vi "Scroller_FGGA_Pump.vi"() -> ()   [LabVIEW 2014]
uses:
  <vilib>/Instr/_visa.llb/VISA Set IO Buffer Mask.ctl
  <vilib>/Instr/_visa.llb/VISA Configure Serial Port (Instr).vi
panel:
  out "element":string
  out "Measured Motor Power (W)":dbl(knob) scale=0.0..800.0
  out "Measured Link Voltage (V)":dbl(knob) scale=0.0..800.0
  out "Measured Motor Current (A)":dbl(knob) scale=0.0..6.0
  out "Pump Controller Temperature":i32(slide) scale=0.0..100.0
  out "Pump Temperature":i32(slide) scale=-500.0..100.0
  in  "Standby Speed threshold":u32(slide) scale=66.0..100.0
  out "Array":string[](array[string])
  in  "Normal Speed threshold":u32(slide) scale=50.0..100.0
  out "running?":bool
  out "Loop Count":i32
  out "Fault register":bool[](array[boolean])
  out "Warning register":bool[](array[boolean])
  out "System status register 2":bool[](array[boolean])
  out "System status register":bool[](array[boolean])
  out "Motor Frequency":i32(graph)
  in  "Set AutoRun":bool
  in  "stop":bool
  in  "Use Standby Speed":bool
  out "error out":errorcluster
  out "Data Out":string
  in  "VISA resource name":refnum<visa-resource-name>="ASRL10::INSTR"
  in  "Pump On/Off":bool
  # "Power limit is active"
  # "Stop command received and pump is stopping"
  # "Acceleration is limited"
  # "Accelerating / running"
  # "Standby Active"
  # "Deceleration is limited"
  # "Above normal speed"
  # "Operating above the ramp speed threshold"
  # "Operating above the overload speed threshold"
  # "Warning Condition"
  # "Control mode"
  # "Fault Condition"
  # "Serial enable active"
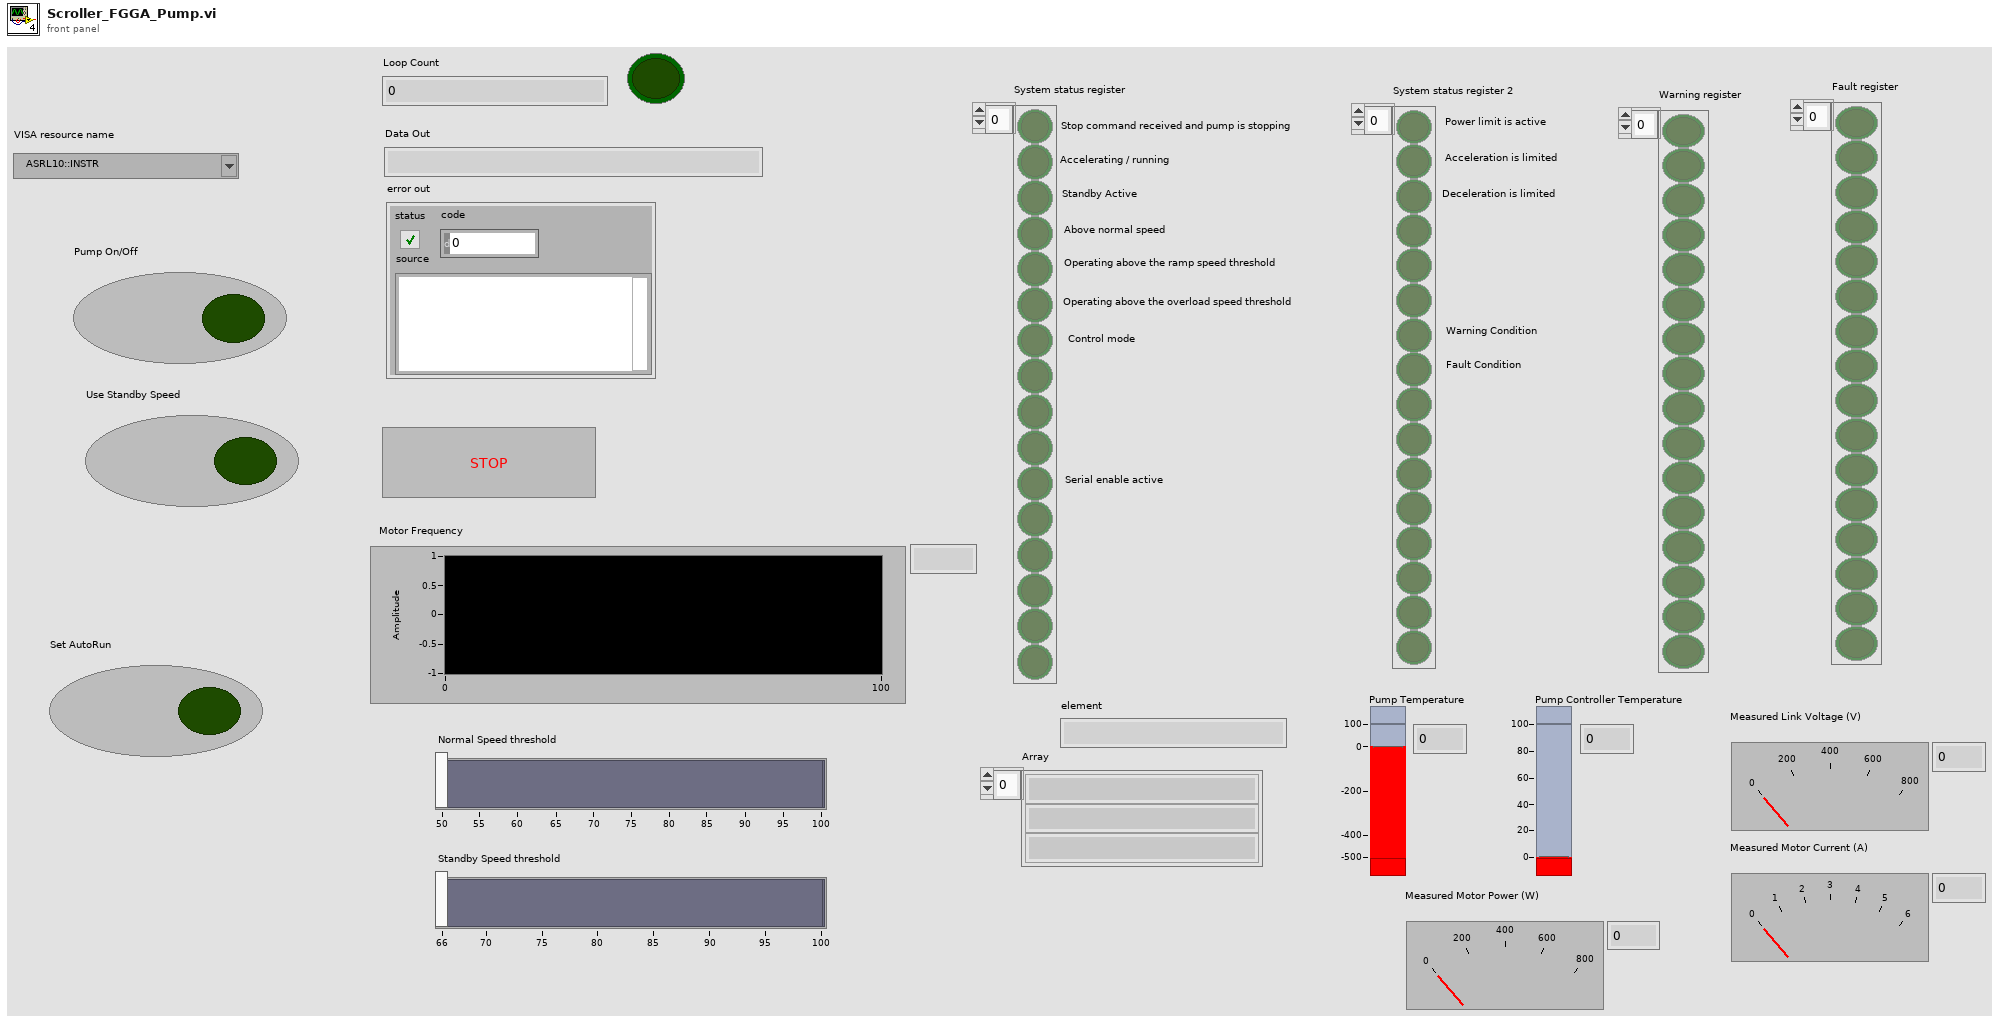
[diagram p1: front panel]
types:
  T1 = typedef "VISA Set IO Buffer Mask.ctl" = u16
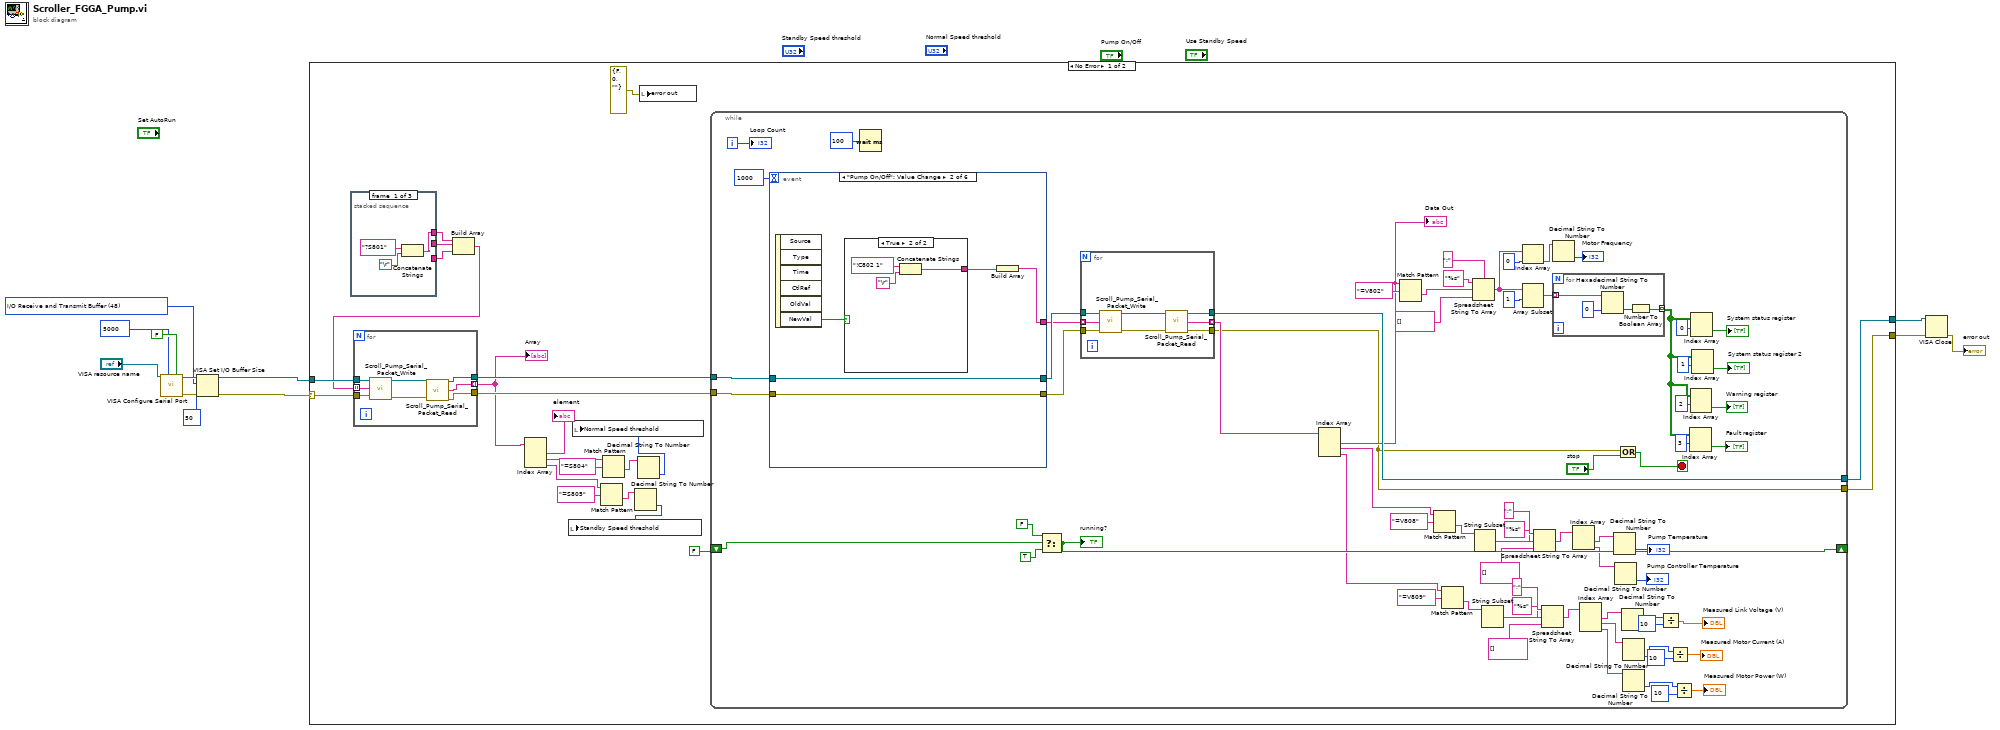
[diagram p0: block diagram]
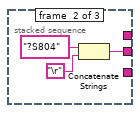
[diagram p2: hidden frame]
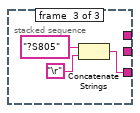
[diagram p3: hidden frame]
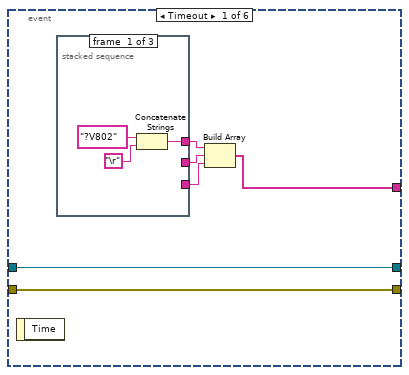
[diagram p4: hidden frame]
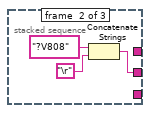
[diagram p5: hidden frame]
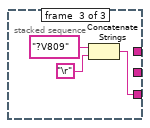
[diagram p6: hidden frame]
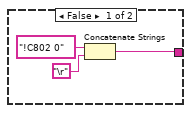
[diagram p7: hidden frame]
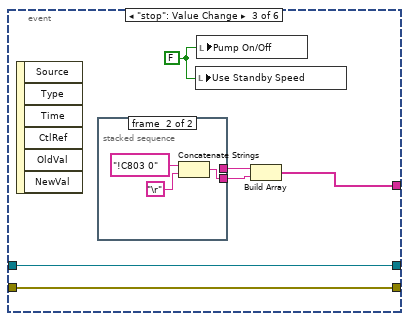
[diagram p8: hidden frame]
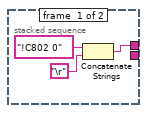
[diagram p9: hidden frame]
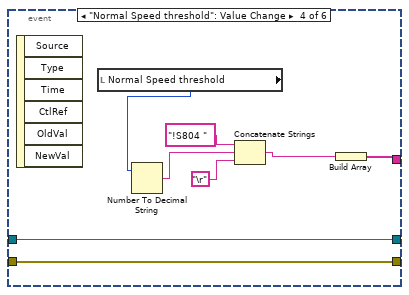
[diagram p10: hidden frame]
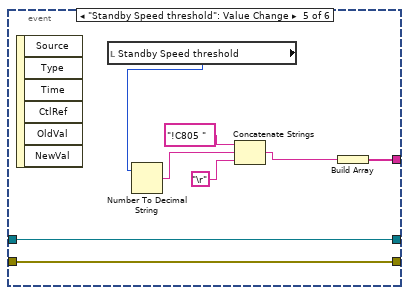
[diagram p11: hidden frame]
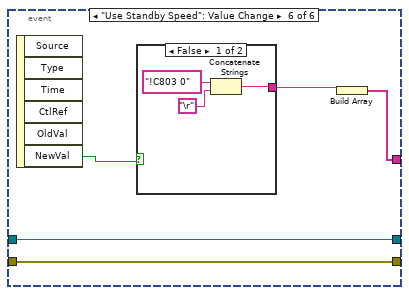
[diagram p12: hidden frame]
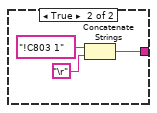
[diagram p13: hidden frame]
diagram:
  w8 = T1 48 items=["I/O Receive Buffer"=16, "I/O Transmit Buffer"=32, "I/O Receive and Transmit Buffer"=48] ("Mask")
  n1 = call-poly "VISA Configure Serial Port"("VISA resource name"="VISA resource name", "timeout (10sec)"=u32 5000, "Enable Termination\nChar (T)"=FALSE ("Enable Termination\nChar (T)")) -> ("VISA resource name out"=w9:refnum<visa-resource-name>, "error out"=w10:errorcluster)  [unwired: 11 in]
  n2 = VISA Set I/O Buffer Size(VISA resource name=w9, mask (16)=w8, size (4096)=u32 50, error in (no error)=w10) -> (VISA resource name out=w2:refnum<visa-resource-name>, error out=w1:errorcluster)
  n3 = case shown="No Error" w1 {
    selector: w1 -> [w32 w199]
    tunnel: w2 -> [w33 w200]
    tunnel: [w29 w200] -> w5
    tunnel: [w28 w199] -> w4
    frame No Error {
      n4 = stacked-sequence {
        tunnel: [_ w46 _] -> w26
        tunnel: [_ _ w49] -> w25
        tunnel: [w43 _ _] -> w23
        frame #0 {
          n5 = Concatenate Strings("?S801" ("string"), "\r") -> (w43:string)
        }
        frame #1 {
          n6 = Concatenate Strings("?S804" ("string"), "\r") -> (w46:string)
        }
        frame #2 {
          n7 = Concatenate Strings("?S805" ("string"), "\r") -> (w49:string)
        }
      }
      n8 = Build Array(w23, w26, w25) -> (w24:string[])
      n9 = for {
        tunnel: w33 -> [w42]
        tunnel: w32 -> [w41]
        tunnel: w24 -> [w40] mode=indexing
        tunnel: [w39] -> w31
        tunnel: [w38] -> w30
        tunnel: [w37] -> w17 mode=indexing
        n10 = call "Scroll_Pump_Serial_Packet_Write.vi"("VISA resource name In"=w42, "Data in"=w40, "error in (no error)"=w41) -> ("VISA resource name Out"=w36:refnum<visa-resource-name>, "error out"=w35:errorcluster)  [unwired: 11 in]
        n11 = call "Scroll_Pump_Serial_Packet_Read.vi"("VISA resource In"=w36, "error in"=w35) -> ("VISA resource Out"=w38:refnum<visa-resource-name>, "Data Out"=w37:string, "error out"=w39:errorcluster)  [unwired: 11 in]
      }
      "Array" <- w17
      n12 = Index Array(array=w17) -> (element #1=→"element":string, element #2=w22:string, element #3=w19:string)  [unwired: 3 in]
      n13 = Match Pattern(string=w19, regular expression="=S805") -> (after substring=w16:string)  [unwired: 1 in, 3 out]
      n14 = Match Pattern(string=w22, regular expression="=S804") -> (after substring=w18:string)  [unwired: 1 in, 3 out]
      n15 = Decimal String To Number(string=w16) -> (number=w14:i32)  [unwired: 2 in, 1 out]
      n16 = local write "Standby Speed threshold"(w14) -> ()
      n17 = Decimal String To Number(string=w18) -> (number=w15:i32)  [unwired: 2 in, 1 out]
      n18 = local write "Normal Speed threshold"(w15) -> ()
      n19 = local write "error out"(errorcluster {"status"=FALSE, "code"=0, "source"=""} ("error out 2")) -> ()
      n20 = while {
        shift-right: [w114] -> _
        shift-left: FALSE -> [w117]
        tunnel: w31 -> [w113]
        tunnel: w30 -> [w112]
        tunnel: [w111] -> w29
        tunnel: [w54] -> w28
        i -> [w118]
        stop <- w53 stop-if-true
        n21 = event shown="[1] \"Pump On/Off\": Value Change" {
          selector: _ -> [_ _ _ _ _ _]
          dyn-events: _ -> [_ _ _ _ _ _]
          timeout: 1000 -> [_ _ _ _ _ _]
          tunnel: [w138 w151 w161 w175 w184 w190] -> w120
          tunnel: [w137 w152 w160 w174 w183 w191] -> w119
          tunnel: w113 -> [w137 w152 w160 w174 w183 w191]
          tunnel: w112 -> [w138 w151 w161 w175 w184 w190]
          tunnel: [w139 w149 w162 w172 w180 w188] -> w60
          event Timeout {
            n22 = event-data() -> ()  [unwired: 1 in, 1 out]
            n23 = stacked-sequence {
              tunnel: [w140 _ _] -> w136
              tunnel: [_ w143 _] -> w135
              tunnel: [_ _ w146] -> w134
              frame #0 {
                n24 = Concatenate Strings("?V802" ("string"), "\r") -> (w140:string)
              }
              frame #1 {
                n25 = Concatenate Strings("?V808" ("string"), "\r") -> (w143:string)
              }
              frame #2 {
                n26 = Concatenate Strings("?V809" ("string"), "\r") -> (w146:string)
              }
            }
            n27 = Build Array(w136, w135, w134) -> (w139:string[])
          }
          event "Pump On/Off": Value Change {
            n28 = event-data() -> ("NewVal"=w153:bool)  [unwired: 1 in, 5 out]
            n29 = case shown="True" w153 {
              tunnel: [w154 w157] -> w150
              frame False {
                n30 = Concatenate Strings("!C802 0" ("string"), "\r") -> (w154:string)
              }
              frame True {
                n31 = Concatenate Strings("!C802 1" ("string"), "\r") -> (w157:string)
              }
            }
            n32 = Build Array(w150) -> (w149:string[])
          }
          event "stop": Value Change {
            w165 = FALSE
            n33 = event-data() -> ()  [unwired: 1 in, 6 out]
            n34 = stacked-sequence {
              tunnel: [w166 _] -> w164
              tunnel: [_ w169] -> w163
              frame #0 {
                n35 = Concatenate Strings("!C802 0" ("string"), "\r") -> (w166:string)
              }
              frame #1 {
                n36 = Concatenate Strings("!C803 0" ("string"), "\r") -> (w169:string)
              }
            }
            n37 = local write "Use Standby Speed"(w165) -> ()
            n38 = local write "Pump On/Off"(w165) -> ()
            n39 = Build Array(w164, w163) -> (w162:string[])
          }
          event "Normal Speed threshold": Value Change {
            n40 = event-data() -> ()  [unwired: 1 in, 6 out]
            n41 = local read "Normal Speed threshold"() -> (w177:u32)
            n42 = Number To Decimal String(number=w177) -> (decimal integer string=w176:string)  [unwired: 1 in]
            n43 = Concatenate Strings("!S804 " ("string"), w176, "\r") -> (w173:string)
            n44 = Build Array(w173) -> (w172:string[])
          }
          event "Standby Speed threshold": Value Change {
            n45 = event-data() -> ()  [unwired: 1 in, 6 out]
            n46 = local read "Standby Speed threshold"() -> (w182:u32)
            n47 = Number To Decimal String(number=w182) -> (decimal integer string=w185:string)  [unwired: 1 in]
            n48 = Concatenate Strings("!C805 " ("string"), w185, "\r") -> (w181:string)
            n49 = Build Array(w181) -> (w180:string[])
          }
          event "Use Standby Speed": Value Change {
            n50 = event-data() -> ("NewVal"=w192:bool)  [unwired: 1 in, 5 out]
            n51 = case shown="False" w192 {
              tunnel: [w193 w196] -> w189
              frame False {
                n52 = Concatenate Strings("!C803 0" ("string"), "\r") -> (w193:string)
              }
              frame True {
                n53 = Concatenate Strings("!C803 1" ("string"), "\r") -> (w196:string)
              }
            }
            n54 = Build Array(w189) -> (w188:string[])
          }
        }
        n55 = Wait (ms)(milliseconds to wait=u32 100) -> ()  [unwired: 1 out]
        n56 = Select(t=FALSE, s=w117, f=TRUE) -> (s? t:f=w114:bool)
        "running?" <- w114
        n57 = for {
          tunnel: [w127] -> w59 mode=indexing
          tunnel: w120 -> [w125]
          tunnel: [w129] -> w111
          tunnel: w119 -> [w124]
          tunnel: [w128] -> w54
          tunnel: w60 -> [w126] mode=indexing
          n58 = call "Scroll_Pump_Serial_Packet_Write.vi"("VISA resource name In"=w125, "Data in"=w126, "error in (no error)"=w124) -> ("VISA resource name Out"=w123:refnum<visa-resource-name>, "error out"=w122:errorcluster)  [unwired: 11 in]
          n59 = call "Scroll_Pump_Serial_Packet_Read.vi"("VISA resource In"=w123, "error in"=w122) -> ("VISA resource Out"=w129:refnum<visa-resource-name>, "Data Out"=w127:string, "error out"=w128:errorcluster)  [unwired: 11 in]
        }
        n60 = Index Array(array=w59) -> (element #1=w56:string, element #2=w57:string, element #3=w58:string)  [unwired: 3 in]
        "Data Out" <- w56
        n61 = Match Pattern(string=w56, regular expression="=V802") -> (after substring=w61:string)  [unwired: 1 in, 3 out]
        n62 = Match Pattern(string=w57, regular expression="=V808") -> (after substring=w105:string)  [unwired: 1 in, 3 out]
        n63 = Match Pattern(string=w58, regular expression="=V809") -> (after substring=w94:string)  [unwired: 1 in, 3 out]
        n64 = Spreadsheet String To Array(delimiter (Tab)=";", format string="%s", spreadsheet string=w61, array type (2D Dbl)=string[] []) -> (array=w75:string[])
        n65 = String Subset(string=w105) -> (substring=w107:string)  [unwired: 2 in]
        n66 = String Subset(string=w94) -> (substring=w96:string)  [unwired: 2 in]
        n67 = Index Array(array=w75, index=0) -> (element=w73:string)
        n68 = Array Subset(array=w75, index=1) -> (w76:string[])  [unwired: 1 in]
        n69 = Spreadsheet String To Array(delimiter (Tab)=";", format string="%s", spreadsheet string=w107, array type (2D Dbl)=string[] []) -> (array=w104:string[])
        n70 = Spreadsheet String To Array(delimiter (Tab)=";", format string="%s", spreadsheet string=w96, array type (2D Dbl)=string[] []) -> (array=w93:string[])
        n71 = Decimal String To Number(string=w73) -> (number=→"Motor Frequency":i32)  [unwired: 2 in, 1 out]
        n72 = for {
          tunnel: w76 -> [w133] mode=indexing
          tunnel: [w130] -> w63 mode=indexing
          n73 = Hexadecimal String To Number(string=w133, default (0uL)=u16 0 ("default (0 U32)")) -> (number=w131:u16)  [unwired: 1 in, 1 out]
          n74 = Number To Boolean Array(number=w131) -> (Boolean array=w130:bool[])
        }
        n75 = Index Array(array=w104) -> (element #1=w103:string, element #2=w101:string)  [unwired: 2 in]
        n76 = Index Array(array=w93) -> (element #1=w92:string, element #2=w91:string, element #3=w90:string)  [unwired: 3 in]
        n77 = Decimal String To Number(string=w103) -> (number=→"Pump Temperature":i32)  [unwired: 2 in, 1 out]
        n78 = Decimal String To Number(string=w101) -> (number=→"Pump Controller Temperature":i32)  [unwired: 2 in, 1 out]
        n79 = Or(x=w54, y="stop") -> (x .or. y?=w53:bool)
        n80 = Decimal String To Number(string=w92) -> (number=w89:i32)  [unwired: 2 in, 1 out]
        n81 = Decimal String To Number(string=w91) -> (number=w85:i32)  [unwired: 2 in, 1 out]
        n82 = Decimal String To Number(string=w90) -> (number=w82:i32)  [unwired: 2 in, 1 out]
        n83 = Divide(x=w89, y=10) -> (x/y=→"Measured Link Voltage (V)":dbl)
        n84 = Divide(x=w85, y=10) -> (x/y=→"Measured Motor Current (A)":dbl)
        n85 = Divide(x=w82, y=10) -> (x/y=→"Measured Motor Power (W)":dbl)
        n86 = Index Array(array=w63, index (row)=3) -> (element=→"Fault register":bool[])  [unwired: 1 in]
        n87 = Index Array(array=w63, index (row)=2) -> (element=→"Warning register":bool[])  [unwired: 1 in]
        n88 = Index Array(array=w63, index (row)=0) -> (element=→"System status register":bool[])  [unwired: 1 in]
        n89 = Index Array(array=w63, index (row)=1) -> (element=→"System status register 2":bool[])  [unwired: 1 in]
        "Loop Count" <- w118
      }
    }
    frame Error {
    }
  }
  n90 = VISA Close(VISA resource name=w5, error in (no error)=w4) -> (error out=→"error out":errorcluster)
